vi "NIVS.FilterChannels.vi"(8 "error in (no error)":errorcluster, 11 "Cluster in":T1) -> (0 "error out":errorcluster, 3 "Cluster out":T1)   [LabVIEW 2015, in "Station.Execution.lvlib"]
uses:
  Station.Execution.lvlib
  Types/Main.StateVariables.ctl
  Types/Execute.UserEventRefs.ctl
  <vilib>/NI Veristand/Execution/Workspace/SystemStateRegEventRef.ctl
  <vilib>/NI Veristand/Execution/Workspace/Target State Info.ctl
  <vilib>/NI Veristand/Execution/Workspace/Target State.ctl
  <vilib>/NI Veristand/Execution/WaveformStreaming/Waveform Data Watcher Event Data (DBL).ctl
  <vilib>/NI Veristand/Execution/WaveformStreaming/WaveformStreamSpecification.ctl
  NationalInstruments.VeriStand.ClientAPI
  <vilib>/NI Veristand/Execution/Workspace/SystemStateEventRef.ctl
  <vilib>/NI Veristand/Execution/Workspace/WorkspaceAPI.ctl
  Types/Waveforms.Info.ctl
  <vilib>/NI Veristand/Execution/WaveformStreaming/Registered Waveform Streams Data Event Refnum (DBL).ctl
  <vilib>/NI Veristand/Execution/WaveformStreaming/WaveformDataWatcherDBL.ctl
  <vilib>/NI Veristand/Execution/WaveformStreaming/WaveformStreamingAPI.ctl
  <vilib>/Utility/miscctls.llb/LVPositionTypeDef.ctl
  Types/UI.Object.ctl
  NationalInstruments.VeriStand
  <vilib>/NI Veristand/Execution/Workspace/NI_VS Workspace ExecutionAPI.lvlib
  <vilib>/NI Veristand/Execution/WaveformStreaming/NI_VS Waveform Streaming Interface.lvlib
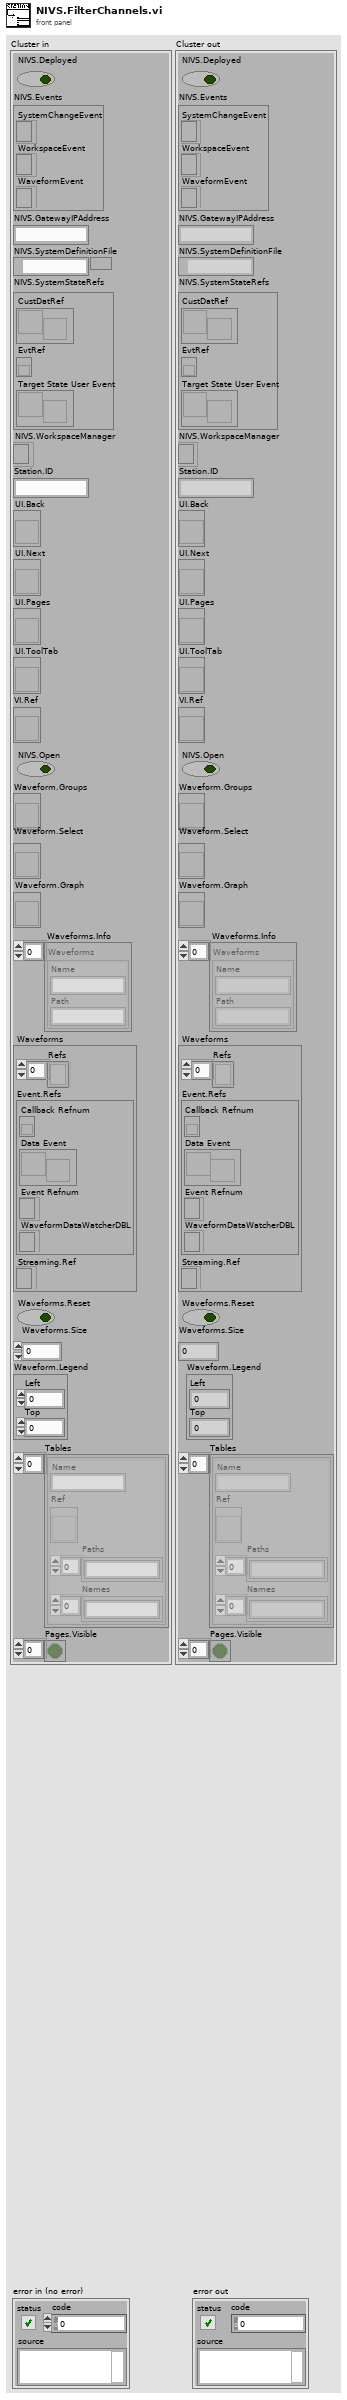
[diagram p1: front panel]
types:
  T1 = typedef "Station.Execution.lvlib/Main.StateVariables.ctl" = cluster{"NIVS.Deployed":bool, "NIVS.Events":T2, "NIVS.GatewayIPAddress":string, "NIVS.SystemDefinitionFile":path, "NIVS.SystemStateRefs":T4, "NIVS.WorkspaceManager":T5, "Station.ID":string, "UI.Back":refnum<vi>, "UI.Next":refnum<vi>, "UI.Pages":refnum<vi>, "UI.ToolTab":refnum<vi>, "VI.Ref":refnum<vi>, "NIVS.Open":bool, "Waveform.Groups":refnum<vi>, "Waveform.Select":refnum<vi>, "Waveform.Graph":refnum<vi>, "Waveforms.Info":T6[], "Waveforms":cluster{"Refs":T7[], "Event.Refs":T8, "Streaming.Ref":T10}, "Waveforms.Reset":bool, "Waveforms.Size":i32, "Waveform.Legend":T11, "Tables":T12[], "Pages.Visible":bool[]}
  T2 = typedef "Station.Execution.lvlib/Execute.UserEventRefs.ctl" = cluster{"SystemChangeEvent":T3, "WorkspaceEvent":refnum<event-registration>, "WaveformEvent":refnum<event-registration>}
  T3 = typedef "NI_VS Workspace ExecutionAPI.lvlib/SystemStateRegEventRef.ctl" = refnum<event-registration>
  T4 = typedef "NI_VS Workspace ExecutionAPI.lvlib/SystemStateEventRef.ctl" = cluster{"CustDatRef":refnum<user-event>, "EvtRef":refnum<k27>, "Target State User Event":refnum<user-event>}
  T5 = typedef "NI_VS Workspace ExecutionAPI.lvlib/WorkspaceAPI.ctl" = refnum<k24>
  T6 = typedef "Station.Execution.lvlib/Waveforms.Info.ctl" = cluster{"Name":string, "Path":string}
  T7 = typedef "NI_VS Waveform Streaming Interface.lvlib/WaveformStreamSpecification.ctl" = refnum<k24>
  T8 = typedef "NI_VS Waveform Streaming Interface.lvlib/Registered Waveform Streams Data Event Refnum (DBL).ctl" = cluster{"Callback Refnum":refnum<k27>, "Data Event":refnum<user-event>, "Event Refnum":refnum<event-registration>, "WaveformDataWatcherDBL":T9}
  T9 = typedef "NI_VS Waveform Streaming Interface.lvlib/WaveformDataWatcherDBL.ctl" = refnum<k24>
  T10 = typedef "NI_VS Waveform Streaming Interface.lvlib/WaveformStreamingAPI.ctl" = refnum<k24>
  T11 = typedef "LVPositionTypeDef.ctl" = cluster{"Left":i32, "Top":i32}
  T12 = typedef "Station.Execution.lvlib/UI.Object.ctl" = cluster{"Name":string, "Ref":refnum<vi>, "Paths":string[], "Names":string[]}
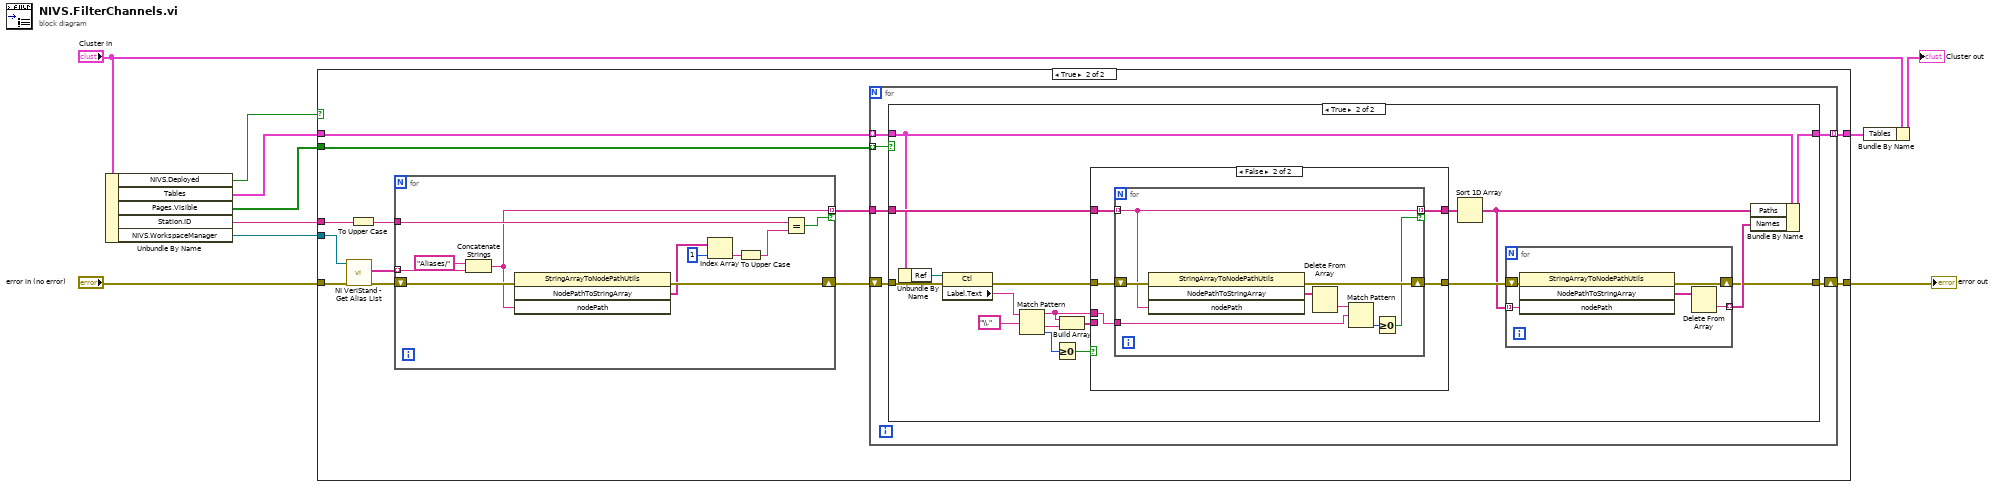
[diagram p0: block diagram]
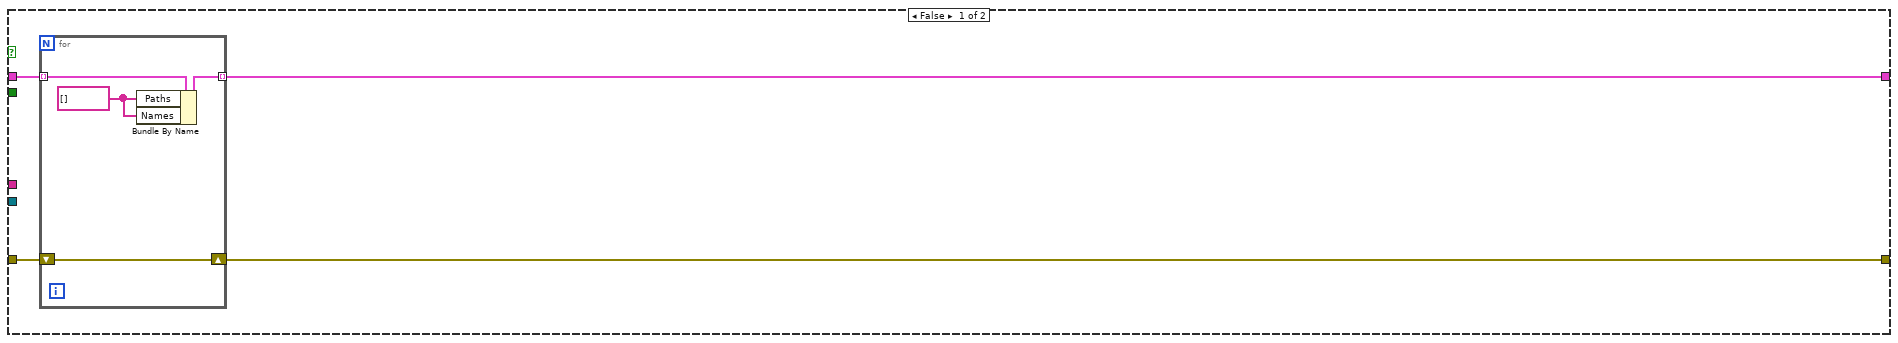
[diagram p2: hidden frame]
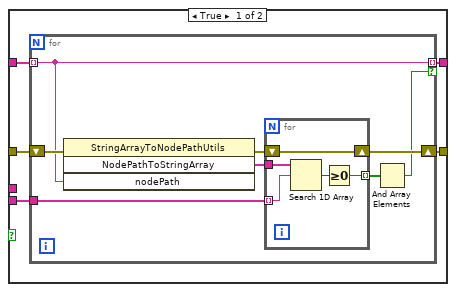
[diagram p4: hidden frame]
diagram:
  n1 = Unbundle By Name("Cluster in") -> ("NIVS.Deployed"=w5:bool, "Tables"=w4:T12[], "Pages.Visible"=w1:bool[], "Station.ID"=w7:string, "NIVS.WorkspaceManager"=w8:T5)
  n2 = case shown="True" w5 {
    tunnel: "error in (no error)" -> [w12 w30]
    tunnel: w8 -> [_ w29]
    tunnel: w7 -> [_ w26]
    tunnel: w4 -> [w14 w23]
    tunnel: [w11 w21] -> w6
    tunnel: [w13 w20] -> w3
    tunnel: w1 -> [_ w19]
    frame False {
      n3 = for {
        shift-right: [w15] -> w11
        shift-left: w12 -> [w15]
        tunnel: w14 -> [w17] mode=indexing
        tunnel: [w16] -> w13 mode=indexing
        w18 = string[] [] ("Channels")
        n4 = Bundle By Name(cluster=w17, "Paths"=w18, "Names"=w18) -> (w16:T12)
      }
    }
    frame True {
      n5 = call <vilib>:"NI VeriStand - Get Alias List.vi"("error in (no error)"=w30, "WorkspaceManager in"=w29) -> ("error out"=w27:errorcluster, "Aliases"=w28:string[])  [unwired: 6 in, 2 out]
      n6 = To Upper Case(1:w26) -> (0:w25:string)
      n7 = for {
        tunnel: w28 -> [w95] mode=indexing
        shift-right: [w97] -> w22
        shift-left: w27 -> [w103]
        tunnel: w25 -> [w99]
        tunnel: [w94] -> w24 mode=indexing if=w98
        n8 = Concatenate Strings("Aliases/", w95) -> (w94:string)
        n9 = invoke class="StringArrayToNodePathUtils" method="NodePathToStringArray"(error in=w103, "nodePath"=w94) -> (error out=w97:errorcluster, "NodePathToStringArray"=w96:string[])  [unwired: 2 in, 2 out]
        n10 = Index Array(array=w96, index=1) -> (element=w101:string)
        n11 = To Upper Case(1:w101) -> (0:w100:string)
        n12 = Equal?(x=w99, y=w100) -> (x = y?=w98:bool)
      }
      n13 = for {
        tunnel: w24 -> [w36]
        shift-right: [w33] -> w21
        shift-left: w22 -> [w34]
        tunnel: w23 -> [w35] mode=indexing
        tunnel: [w32] -> w20 mode=indexing
        tunnel: w19 -> [w31] mode=indexing
        n14 = case shown="True" w31 {
          tunnel: w36 -> [_ w52]
          tunnel: w35 -> [w38 w42]
          tunnel: w34 -> [w37 w41]
          tunnel: [w37 w40] -> w33
          tunnel: [w38 w39] -> w32
          frame False {
          }
          frame True {
            n15 = Unbundle By Name(w42) -> ("Ref"=w56:refnum<vi>)
            n16 = property class="Ctl"(reference=w56, error in=w41) -> (error out=w51:errorcluster, "Label.Text"=w49:string)  [unwired: 1 out]
            n17 = Match Pattern(string=w49, regular expression="\\.") -> (before substring=w46:string, after substring=w53:string, offset past match=w54:i32)  [unwired: 1 in, 1 out]
            n18 = Greater Or Equal To 0?(x=w54) -> (x >= 0?=w48:bool)
            n19 = Build Array(w46, w53) -> (w47:string[])
            n20 = case shown="False" w48 {
              tunnel: w52 -> [w61 w79]
              tunnel: w51 -> [w60 w78]
              tunnel: w47 -> [w59 _]
              tunnel: [w58 w77] -> w50
              tunnel: [w57 w76] -> w44
              tunnel: w46 -> [_ w75]
              frame True {
                n21 = for {
                  tunnel: w61 -> [w63] mode=indexing
                  shift-right: [w64] -> w57
                  shift-left: w60 -> [w69]
                  tunnel: w59 -> [w67]
                  tunnel: [w63] -> w58 mode=indexing if=w62
                  n22 = invoke class="StringArrayToNodePathUtils" method="NodePathToStringArray"(error in=w69, "nodePath"=w63) -> (error out=w66:errorcluster, "NodePathToStringArray"=w68:string[])  [unwired: 2 in, 2 out]
                  n23 = for {
                    tunnel: w68 -> [w74]
                    tunnel: w67 -> [w73] mode=indexing
                    shift-right: [w71] -> w64
                    shift-left: w66 -> [w71]
                    tunnel: [w70] -> w65 mode=indexing
                    n24 = Search 1D Array(1D array=w74, element=w73) -> (index of element=w72:i32)  [unwired: 1 in]
                    n25 = Greater Or Equal To 0?(x=w72) -> (x >= 0?=w70:bool)
                  }
                  n26 = And Array Elements(Boolean array=w65) -> (logical AND=w62:bool)
                }
              }
              frame False {
                n27 = for {
                  tunnel: w79 -> [w83] mode=indexing
                  shift-right: [w84] -> w76
                  shift-left: w78 -> [w87]
                  tunnel: w75 -> [w85]
                  tunnel: [w83] -> w77 mode=indexing if=w80
                  n28 = invoke class="StringArrayToNodePathUtils" method="NodePathToStringArray"(error in=w87, "nodePath"=w83) -> (error out=w84:errorcluster, "NodePathToStringArray"=w86:string[])  [unwired: 2 in, 2 out]
                  n29 = Delete From Array(array=w86) -> (deleted portion=w82:string)  [unwired: 2 in, 1 out]
                  n30 = Match Pattern(string=w82, regular expression=w85) -> (offset past match=w81:i32)  [unwired: 1 in, 3 out]
                  n31 = Greater Or Equal To 0?(x=w81) -> (x >= 0?=w80:bool)
                }
              }
            }
            n32 = Sort 1D Array(array=w50) -> (sorted array=w43:string[])
            n33 = for {
              tunnel: [w91] -> w45 mode=indexing
              shift-right: [w89] -> w40
              shift-left: w44 -> [w90]
              tunnel: w43 -> [w88] mode=indexing
              n34 = invoke class="StringArrayToNodePathUtils" method="NodePathToStringArray"(error in=w90, "nodePath"=w88) -> (error out=w89:errorcluster, "NodePathToStringArray"=w92:string[])  [unwired: 2 in, 2 out]
              n35 = Delete From Array(array=w92) -> (deleted portion=w91:string)  [unwired: 2 in, 1 out]
            }
            n36 = Bundle By Name(cluster=w42, "Paths"=w43, "Names"=w45) -> (w39:T12)
          }
        }
      }
    }
  }
  "error out" <- w6
  n37 = Bundle By Name(cluster="Cluster in", "Tables"=w3) -> (→"Cluster out":T1)
